vi "CalculateFreq.vi"(8 "error in (no error)":errorcluster, 11 "voltage waveforms":waveform(dbl)[](array[waveform])) -> (0 "error out":errorcluster, 3 "frequency":dbl=60.0)   [LabVIEW 2016, in "McsaAnalysisFunctions.lvlib"]
uses:
  <vilib>/addons/InsightCM/Utilities/Analysis/MCSA/McsaAnalysisFunctions.lvlib
  <vilib>/addons/Electrical Power/Basic/NI_EP_Basic.lvlib
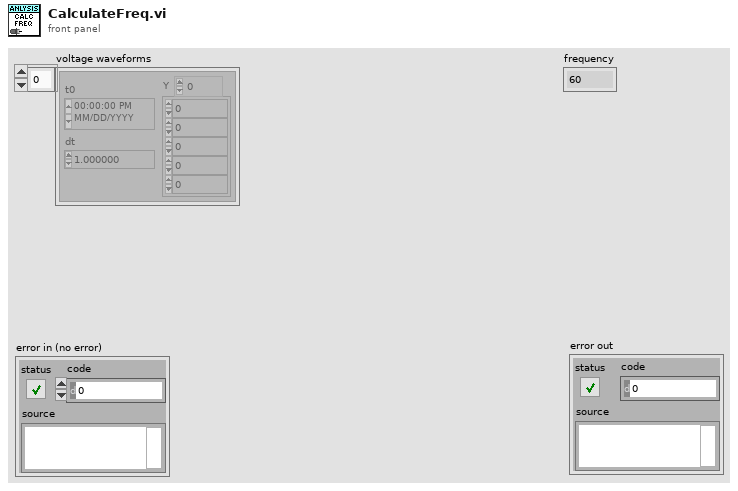
[diagram p1: front panel]
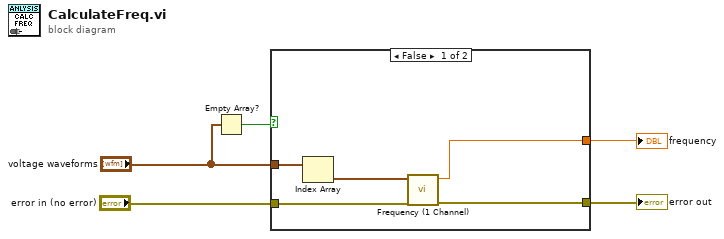
[diagram p0: block diagram]
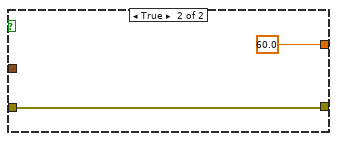
[diagram p2: hidden frame]
diagram:
  n1 = Empty Array?(array="voltage waveforms") -> (empty?=w3:bool)
  n2 = case shown="False" w3 {
    tunnel: [w8 60.0 ("frequency")] -> w5
    tunnel: [w10 w12] -> w4
    tunnel: "voltage waveforms" -> [w9 _]
    tunnel: "error in (no error)" -> [w7 w12]
    frame False {
      n3 = Index Array(array=w9) -> (element=w6:waveform(dbl))  [unwired: 1 in]
      n4 = call <vilib>:"Frequency (1 Channel).vi"("error in (no error)"=w7, "waveform"=w6) -> ("error out"=w10:errorcluster, "frequency"=w8:dbl)  [unwired: 8 in]
    }
    frame True {
    }
  }
  "frequency" <- w5
  "error out" <- w4
